vi "Main Chroma 19053 hipot_driver.vi"   [LabVIEW 2020]
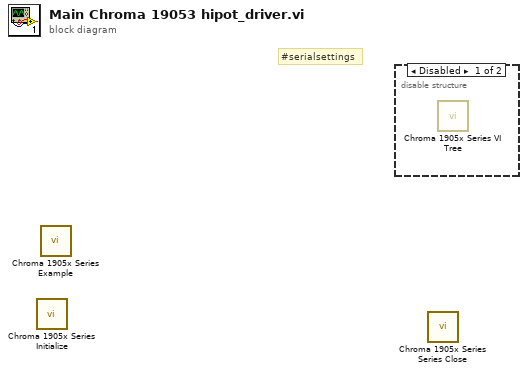
[diagram p0: block diagram]
diagram:
  # "#serialsettings"
  n1 = call <instrlib>:"Chroma 1905x Series Initialize.vi"() -> ()  [unwired: 4 in, 3 out]
  n2 = call <instrlib>:"Chroma 1905x Series Example.vi"() -> ()  [unwired: 1 in]
  n3 = disable-structure shown="Disabled" {
    frame Disabled {
      n4 = call <instrlib>:"Chroma 1905x Series VI Tree.vi"() -> ()  [unwired: 1 in]
    }
    frame Enabled {
    }
  }
  n5 = call <instrlib>:"Chroma 1905x Series Series Close.VI"() -> ()  [unwired: 4 in, 1 out]
